vi "ElementWiseMinus.vi"(9 "a":dbl, 10 "Array [in]":dbl[](array[numeric])) -> (2 "Array[out]":dbl[](array[numeric]))   [LabVIEW 2013]
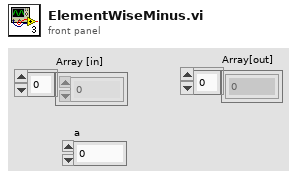
[diagram p1: front panel]
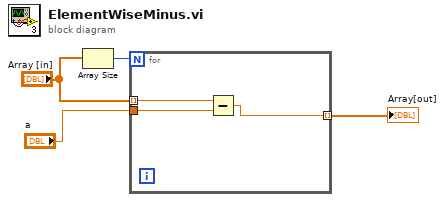
[diagram p0: block diagram]
diagram:
  n1 = Array Size(array="Array [in]") -> (size(s)=w4:i32)
  n2 = for {
    N: w4 -> [_]
    tunnel: "Array [in]" -> [w7] mode=indexing
    tunnel: "a" -> [w6]
    tunnel: [w5] -> w1 mode=indexing
    n3 = Subtract(x=w7, y=w6) -> (x-y=w5:dbl)
  }
  "Array[out]" <- w1
